vi "Set Frequency Mode.vi"(8 "error in (no error)":errorcluster, 10 "Frequency Mode":T1(ring), 11 "VISA resource name":refnum<visa-resource-name>) -> (0 "error out":errorcluster, 3 "VISA resource name out":refnum<visa-resource-name>)   [LabVIEW 2017, in "Agilent PSG MXG Series.lvlib"]
uses:
  Agilent PSG MXG Series.lvlib
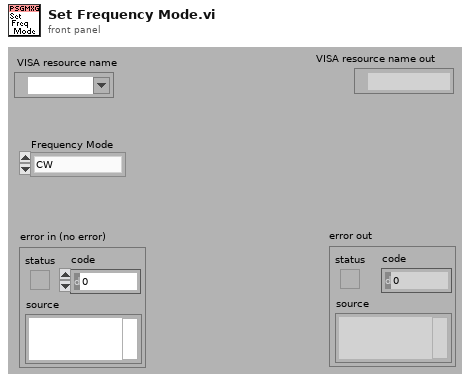
[diagram p1: front panel]
types:
  T1 = enum16{"CW", "Fixed", "Stepped Sweep", "List Sweep"}
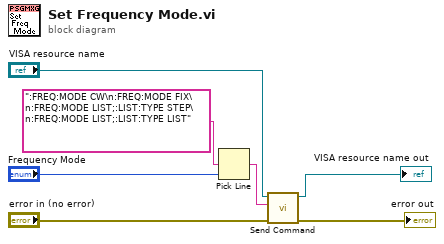
[diagram p0: block diagram]
diagram:
  n1 = Pick Line(multi-line string=":FREQ:MODE CW\n:FREQ:MODE FIX\n:FREQ:MODE LIST;:LIST:TYPE STEP\n:FREQ:MODE LIST;:LIST:TYPE LIST", line index="Frequency Mode") -> (output string=w4:string)  [unwired: 1 out]
  n2 = call "Send Command.vi"("error in (no error)"="error in (no error)", "write buffer"=w4, "VISA resource name"="VISA resource name") -> ("error out"=→"error out":errorcluster, "VISA resource name out"=→"VISA resource name out":refnum<visa-resource-name>)  [unwired: 7 out]
